vi "Measure Data to 2D Format by Cursor.vi"(8 "error in (no error)":errorcluster, 11 "Graph Combined Reference":refnum<vi>) -> (0 "error out":errorcluster, 3 "Graph Combined Reference":refnum<vi>)   [LabVIEW 2023]
panel:
  out "2D String Data":string[][](array[string])
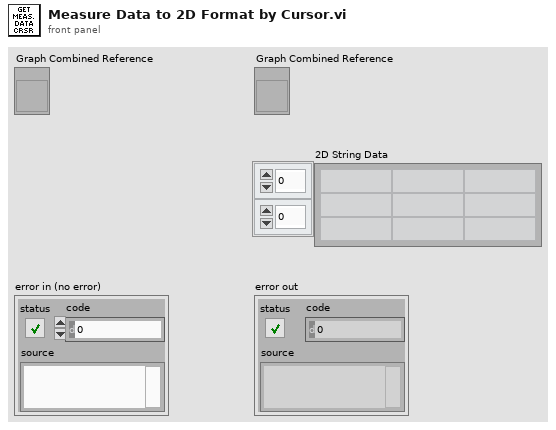
[diagram p1: front panel]
types:
  T1 = cluster{"Load currents":dbl[], "Efficiency":dbl[]}[]
  T2 = typedef "LVCursorListTypeDef.ctl" = cluster{"Name":string, "Color":u32, "Style":u8, "Point Style":u8, "Name Visible":bool, "Allow Drag":bool, "Cursor Mode":u32, "Plot":i32, "Index":i32, "Position":cluster{"X":dbl, "Y":dbl}, "X Scale":u32, "Y Scale":u32, "Watch Plots":i32[], "Watch All Plots":bool, "Plot Area":i32, "Label Offset":cluster{"X":dbl, "Y":dbl}}[]
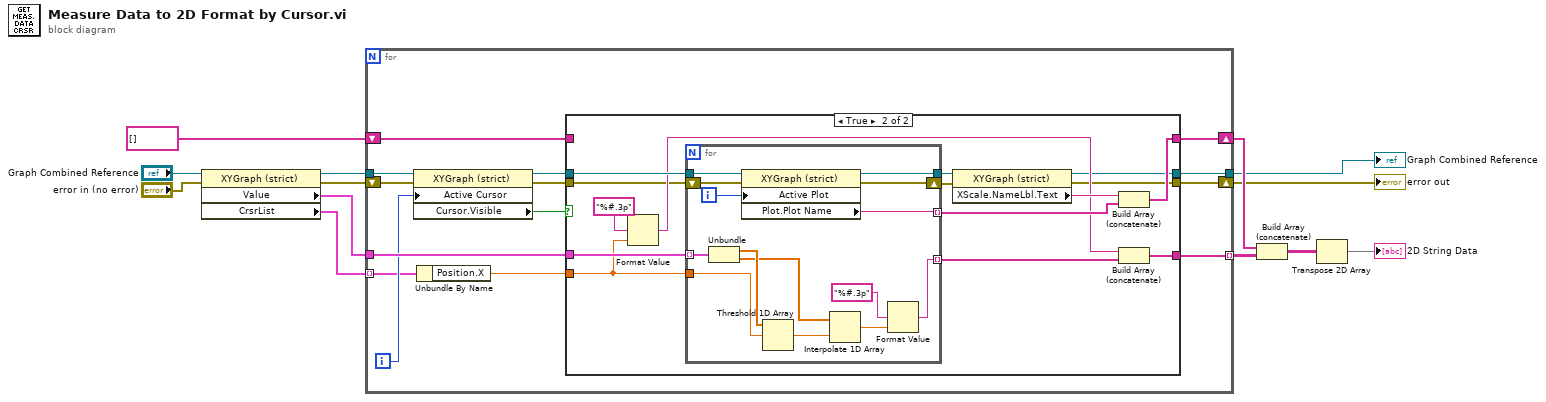
[diagram p0: block diagram]
diagram:
  n1 = property on="Property Node" class="XYGraph (strict)"(reference="Graph Combined Reference", error in="error in (no error)") -> (reference out=w6:refnum<vi>, error out=w4:errorcluster, "Value"=w10:T1, "CrsrList"=w12:T2)
  n2 = for {
    tunnel: w10 -> [w27]
    tunnel: w12 -> [w19] mode=indexing
    tunnel: [w26] -> w8 mode=indexing
    tunnel: w6 -> [w24]
    shift-right: [w25] -> w9
    shift-left: string[] [] -> [w20]
    shift-right: [w15] -> w3
    shift-left: w4 -> [w17]
    tunnel: [w14] -> w2
    i -> [w22]
    n3 = property on="Property Node" class="XYGraph (strict)"(reference=w24, error in=w17, "Active Cursor"=w22) -> (reference out=w23:refnum<vi>, error out=w16:errorcluster, "Cursor.Visible"=w21:bool)
    n4 = Unbundle By Name(w19) -> ("Position.X"=w18:dbl)
    n5 = case shown="True" w21 {
      tunnel: w27 -> [_ w45]
      tunnel: [_ w43] -> w26
      tunnel: [w30 w39] -> w25
      tunnel: w23 -> [w28 w38]
      tunnel: w18 -> [_ w36]
      tunnel: w20 -> [w30 _]
      tunnel: w16 -> [w29 w35]
      tunnel: [w29 w33] -> w15
      tunnel: [w28 w32] -> w14
      frame False {
      }
      frame True {
        n6 = Format Value(format string="%#.3p", value (0)=w36) -> (output string=w37:string)  [unwired: 1 in]
        n7 = for {
          tunnel: [w58] -> w44 mode=indexing
          tunnel: w45 -> [w57] mode=indexing
          tunnel: w36 -> [w54]
          tunnel: [w52] -> w40 mode=indexing
          tunnel: w38 -> [w51]
          tunnel: [w50] -> w42
          shift-right: [w46] -> w34
          shift-left: w35 -> [w47]
          i -> [w53]
          n8 = Unbundle(w57) -> ("Load currents"=w56:dbl[], "Efficiency"=w55:dbl[])
          n9 = property on="Property Node" class="XYGraph (strict)"(reference=w51, error in=w47, "Active Plot"=w53) -> (reference out=w50:refnum<vi>, error out=w46:errorcluster, "Plot.Plot Name"=w52:string)
          n10 = Threshold 1D Array(2:w54, 3:w56) -> (0:w59:dbl)  [unwired: 1 in]
          n11 = Interpolate 1D Array(1:w59, 2:w55) -> (0:w49:dbl)
          n12 = Format Value(format string="%#.3p", value (0)=w49) -> (output string=w58:string)  [unwired: 1 in]
        }
        n13 = property on="Property Node" class="XYGraph (strict)"(reference=w42, error in=w34) -> (reference out=w32:refnum<vi>, error out=w33:errorcluster, "XScale.NameLbl.Text"=w41:string)
        n14 = Build Array (concatenate)(w41, w40) -> (w39:string[])
        n15 = Build Array (concatenate)(w37, w44) -> (w43:string[])
      }
    }
  }
  "Graph Combined Reference" <- w2
  "error out" <- w3
  n16 = Build Array (concatenate)(w9, w8) -> (w7:string[][])
  n17 = Transpose 2D Array(2D array=w7) -> (transposed array=→"2D String Data":string[][])
